vi "FestoCPX.PressureCircuit.Array.vi"(6 "Delay [ms] (0)":u32, 7 "Coils":T2[](array[typedef]), 8 "error in":errorcluster, 11 "Actions":T1[](array[typedef])) -> (0 "error out":errorcluster)   [LabVIEW 2014]
uses:
  FestoCPX.PressureCircuit.Array.ctl
  FestoCPX.PressureCircuit.Array.Actionctl.ctl
  FestoCPX.DO.Signal.ctl
  FestoCPX.DO.Data.States.Set.vi
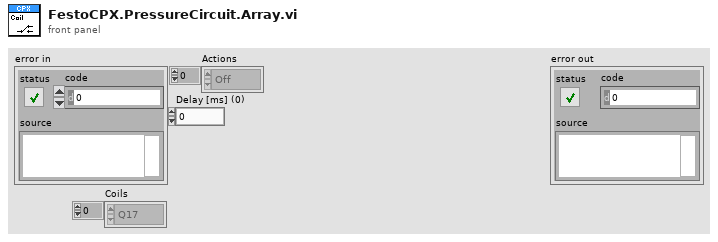
[diagram p1: front panel]
types:
  T1 = typedef "FestoCPX.PressureCircuit.Array.Actionctl.ctl" = enum16{"Off", "k1", "k2"}
  T2 = typedef "FestoCPX.PressureCircuit.Array.ctl" = enum16{"Q17"}
  T3 = typedef "FestoCPX.DO.Signal.ctl" = enum16{"0_0 Start Button LED", "0_1 White Button LED", "0_2 Blue Button LED", "0_3 Red Button LED", "0_4 Safety Circuit Reset", "0_5 Air Main Valve", "0_6 Laser Interlock", "0_7 SPARE", "1_0 SPARE", "1_1 Traffic Light Red", "1_2 Traffic Light Orange", "1_3 Traffic Light Green", "1_4 Horn 1", "1_5 SPARE", "1_6 SPARE", "1_7 SPARE", "2_0 Vent B Work", "2_1 Vent B Home", "2_2 Vent A Work", "2_3 Vent A Home", "2_4 Product Press A Work", "2_5 Product Press A Home", "2_6 Product Press B Work", "2_7 Product Press B Home", "3_0 Pneumatic Connection A Work", "3_1 Pneumatic Connection A Home", "3_2 Pneumatic Connection B Work", "3_3 Pneumatic Connection B Home", "3_4 Laser Press Work", "3_5 Laser Press Home", "5_0 Table Turn Work", "5_1 Table Turn Home"}
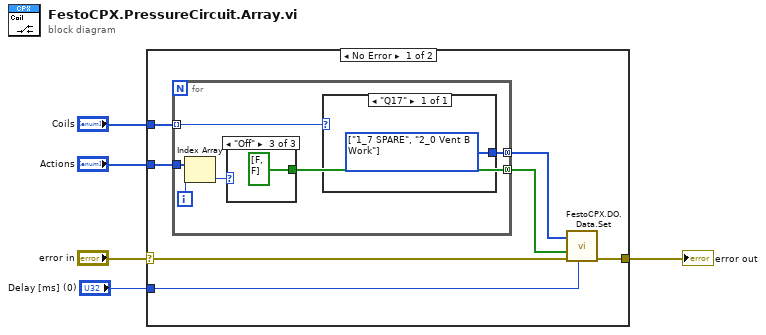
[diagram p0: block diagram]
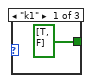
[diagram p2: hidden frame]
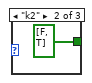
[diagram p3: hidden frame]
diagram:
  n1 = case shown="No Error" "error in" {
    selector: "error in" -> [w12 w23]
    tunnel: [w11 w23] -> w4
    tunnel: "Coils" -> [w10 _]
    tunnel: "Actions" -> [w9 _]
    tunnel: "Delay [ms] (0)" -> [w6 _]
    frame No Error {
      n2 = for {
        tunnel: w10 -> [w18] mode=indexing
        tunnel: w9 -> [w15]
        tunnel: [w17] -> w8 mode=concatenating
        tunnel: [w16] -> w7 mode=concatenating
        i -> [w13]
        n3 = Index Array(array=w15, index=w13) -> (element=w14:T1)
        n4 = case shown="\"Off\"" w14 {
          tunnel: [bool[] [TRUE, FALSE] ("State") bool[] [FALSE, TRUE] ("State") bool[] [FALSE, FALSE] ("State")] -> w16
          frame "k1" {
          }
          frame "k2" {
          }
          frame "Off" {
          }
        }
        n5 = case shown="\"Q17\"" w18 {
          tunnel: [w22] -> w17
          frame "Q17" {
            w22 = T3[] [enum."1_7 SPARE", enum."2_0 Vent B Work"] items=["0_0 Start Button LED", "0_1 White Button LED", "0_2 Blue Button LED", "0_3 Red Button LED", "0_4 Safety Circuit Reset", "0_5 Air Main Valve", "0_6 Laser Interlock", "0_7 SPARE", "1_0 SPARE", "1_1 Traffic Light Red", "1_2 Traffic Light Orange", "1_3 Traffic Light Green", "1_4 Horn 1", "1_5 SPARE", "1_6 SPARE", "1_7 SPARE", "2_0 Vent B Work", "2_1 Vent B Home", "2_2 Vent A Work", "2_3 Vent A Home", "2_4 Product Press A Work", "2_5 Product Press A Home", "2_6 Product Press B Work", "2_7 Product Press B Home", "3_0 Pneumatic Connection A Work", "3_1 Pneumatic Connection A Home", "3_2 Pneumatic Connection B Work", "3_3 Pneumatic Connection B Home", "3_4 Laser Press Work", "3_5 Laser Press Home", "5_0 Table Turn Work", "5_1 Table Turn Home"] ("CPX.DO")
          }
        }
      }
      n6 = call-poly "FestoCPX.DO.Data.Set.vi"("Delay [ms] (0)"=w6, "error in (no error)"=w12, "State"=w7, "CPX.DO"=w8) -> ("error out"=w11:errorcluster)  [unwired: 7 in]
    }
    frame Error {
    }
  }
  "error out" <- w4
